vi "BLED1112_app-connection.vi"(0 "COM Bluegiga in":refnum<visa-resource-name>="COM8", 5 "MAC Address":string="D9:2F:10:92:34:F2", 7 "Address Type":enum16{"Public", "Random"}(ring)=enum."Random", 9 "Conn Try no":i32=5, 11 "error in":errorcluster) -> (4 "COM out":refnum<visa-resource-name>="COM8", 6 "Connection Ok":bool=TRUE, 8 "Device Name":string="JUN_JUN", 10 "Handle table":string[][](array[string])=[["0001", "1800", "2800"], ["0002", "1800", "2803"], ["0003", "1800", "2A00"], ["0004", "1800", "2803"], ["0005", "1800", "2A01"], ["0006", "1800", "2803"], ["0007", "1800", "2A04"], ["0008", "1801", "2800"], ["0009", "0000F00D1212EFDE1523785FEF13D123", "2800"], ["000A", "0000F00D1212EFDE1523785FEF13D123", "2803"], ["000B", "0000F00D1212EFDE1523785FEF13D123", "000000011212EFDE1523785FEF13D123"], ["000C", "0000F00D1212EFDE1523785FEF13D123", "2902"], ["000D", "000000021212EFDE1523785FEF13D123", "2800"], ["000E", "000000021212EFDE1523785FEF13D123", "2803"], ["000F", "000000021212EFDE1523785FEF13D123", "000000021212EFDE1523785FEF13D123"], ["0010", "000000021212EFDE1523785FEF13D123", "2902"]], 14 "Connection Status":T1={"MAC Address"="D9:2F:10:92:34:F2", "cnx handle"=0, "cnx flags"=5, "Address Type"=1, "Connection Interval (ms)"=15, "Timeout(ms)"=1000, "Latency"=0, "bonding handle"=255} {"Address Type" items=["Public", "Random"]}, 15 "에러 출력":errorcluster={"status"=FALSE, "code"=1073676294, "source"="ble_read_message.vi->ble_read_specific_message.vi->ble_evt_attclient_procedue_completed.vi->ble_write_by_handle_uint8array.vi->ble_write_by_service_characteristic_uint8array.vi->BLED1112_app-connection.vi->[BLE Test] ble_read_write_characteristics.vi 안에 VISA 읽기"})   [LabVIEW 2015]
uses:
  Lib_Bled112 toolkit/type_def/connection_status_bundle.ctl
  Lib_Bled112 toolkit/type_def/address_type.ctl
  Lib_Bled112 toolkit/ble_functions/ble_write_by_service_characteristic_uint8array.vi
panel:
  out "Conn try":i32=4
  out "Get Device name?":bool=TRUE
  out "Get handle table?":bool=TRUE
  out "Connected?":bool=TRUE
  # "BLE Connection"
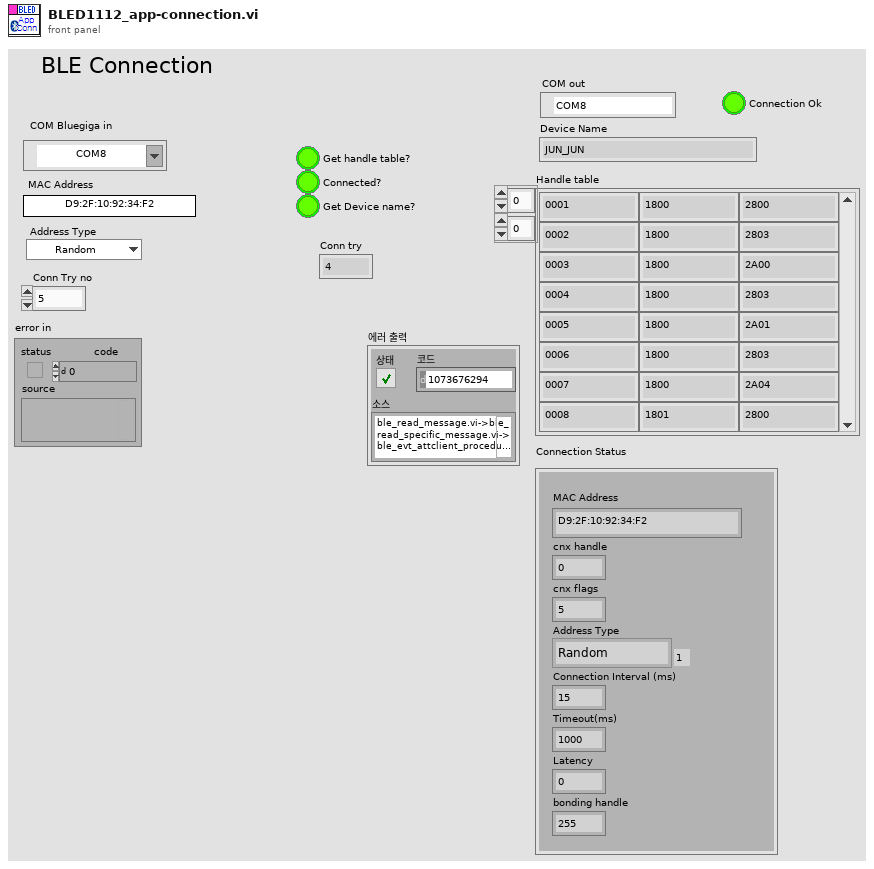
[diagram p1: front panel]
types:
  T1 = typedef "connection_status_bundle.ctl" = cluster{"MAC Address":string, "cnx handle":u8, "cnx flags":u8, "Address Type":T2, "Connection Interval (ms)":u16, "Timeout(ms)":u16, "Latency":u16, "bonding handle":u8}
  T2 = typedef "address_type.ctl" = u8
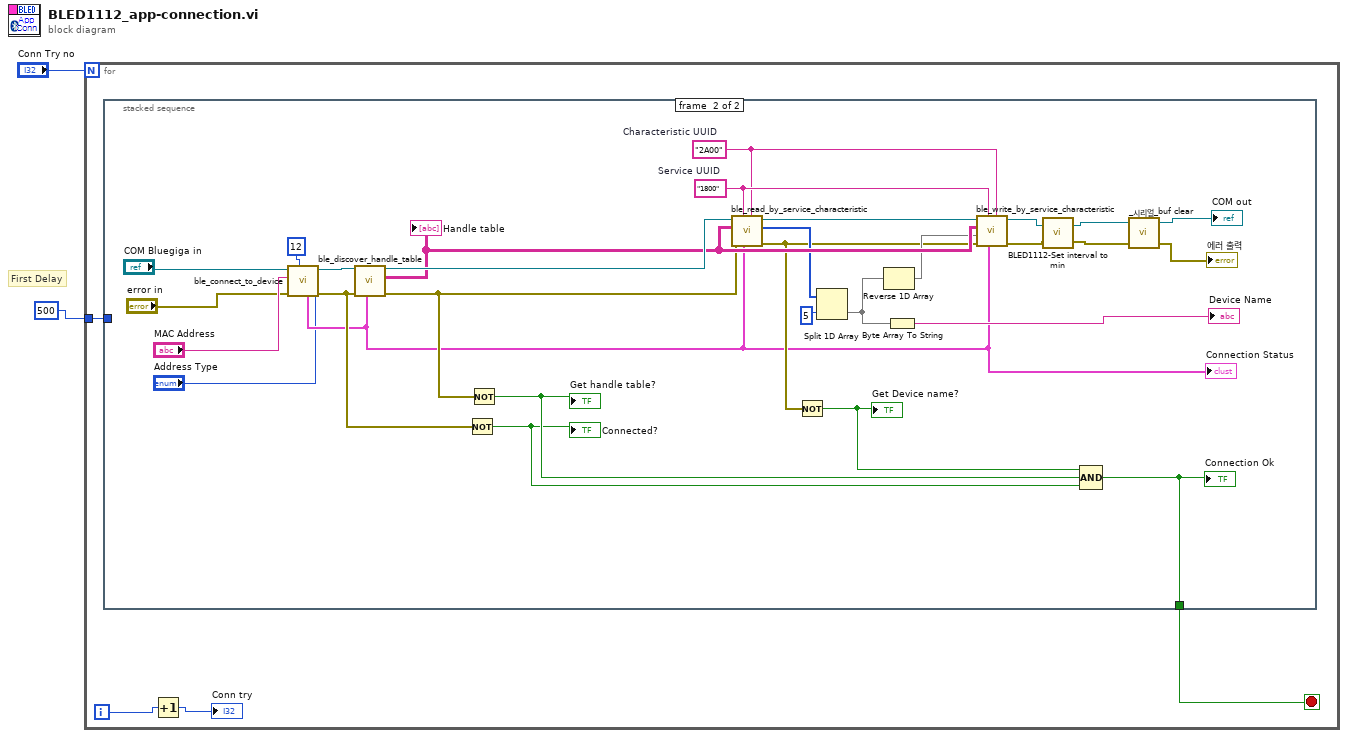
[diagram p0: block diagram]
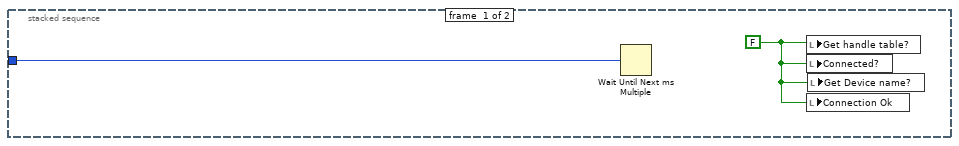
[diagram p2: hidden frame]
diagram:
  # "First Delay"
  n1 = for {
    N: "Conn Try no" -> [_]
    tunnel: u32 500 ("ms 배수") -> [w3]
    i -> [w5]
    stop <- w6 stop-if-true
    n2 = stacked-sequence {
      tunnel: [_ w9] -> w6
      tunnel: w3 -> [w8 _]
      frame #0 {
        w7 = FALSE ("Get handle table?")
        n3 = Wait Until Next ms Multiple(millisecond multiple=w8) -> ()  [unwired: 1 out]
        n4 = local write "Get handle table?"(w7) -> ()
        n5 = local write "Connected?"(w7) -> ()
        n6 = local write "Connection Ok"(w7) -> ()
        n7 = local write "Get Device name?"(w7) -> ()
      }
      frame #1 {
        w33 = "2A00"  # Characteristic UUID
        w34 = "1800"  # Service UUID
        n8 = call "ble_connect_to_device.vi"("Address Type"="Address Type", "Connection Interval Min (75ms)"=u16 12, "error in (no error)"="error in", "MAC Address"="MAC Address", "COM Bluegiga in"="COM Bluegiga in") -> ("error out"=w27:errorcluster, "COM Bluegiga out"=w28:refnum<visa-resource-name>, "Connection Status"=w19:T1)  [unwired: 4 in]
        "Connection Status" <- w19
        n9 = call "ble_discover_handle_table.vi"("Connection Status"=w19, "error in (no error)"=w27, "COM Bluegiga in"=w28) -> ("error out"=w26:errorcluster, "Handle table"=w32:string[][], "COM Bluegiga out"=w38:refnum<visa-resource-name>)  [unwired: 6 in]
        "Handle table" <- w32
        n10 = Not(x=w27) -> (.not. x?=w10:bool)
        "Connected?" <- w10
        n11 = Not(x=w26) -> (.not. x?=w11:bool)
        "Get handle table?" <- w11
        n12 = call "ble_read_by_service_characteristic.vi"("Characteristic UUID"=w33, "Connection Status"=w19, "Service UUID"=w34, "error in (no error)"=w26, "Handle table"=w32, "COM Bluegiga in"=w38) -> ("error out"=w25:errorcluster, "characteristic value"=w31:u8[], "COM Bluegiga out"=w35:refnum<visa-resource-name>)  [unwired: 3 in]
        n13 = Not(x=w25) -> (.not. x?=w12:bool)
        "Get Device name?" <- w12
        n14 = Split 1D Array(array=w31, index=5) -> (second subarray=w30:u8[])  [unwired: 1 out]
        n15 = Reverse 1D Array(array=w30) -> (reversed array=w29:u8[])
        n16 = Byte Array To String(unsigned byte array=w30) -> (string=→"Device Name":string)
        n17 = call-poly "ble_write_by_service_characteristic.vi"("Characteristic UUID"=w33, "Connection Status"=w19, "Service UUID"=w34, "error in (no error)"=w25, "data"=w29, "Handle table"=w32, "COM Bluegiga in"=w35) -> ("error out"=w23:errorcluster, "COM Bluegiga out"=w24:refnum<visa-resource-name>)  [unwired: 3 in]
        n18 = call "BLED1112-Set interval to min.vi"("에러 입력(에러 없음)"=w23, "VISA 리소스 이름"=w24) -> ("에러 출력"=w21:errorcluster, "VISA 리소스 이름 출력"=w22:refnum<visa-resource-name>)
        n19 = Compound Arithmetic op=AND ("복합 연산")(w12, w11, w10) -> (w9:bool)
        "Connection Ok" <- w9
        n20 = call "_시리얼_buf clear.vi"("에러 출력 2"=w21, "시리얼 포트"=w22) -> ("에러 출력"=→"에러 출력":errorcluster, "시리얼 포트 2"=→"COM out":refnum<visa-resource-name>)  [unwired: 2 in]
      }
    }
    n21 = Increment(x=w5) -> (x+1=→"Conn try":i32)
  }
